vi "Get Required Objects.vi"(8 "error in":errorcluster, 11 "Device Profile in":refnum<class "Device Profile.lvclass">) -> (0 "error out":errorcluster, 2 "Required Objects":set{T1}(c389), 3 "Device Profile out":refnum<class "Device Profile.lvclass">)   [LabVIEW 2020, in "CANopen.lvlib" / "Device Profile.lvclass"]
uses:
  Device Profile.lvclass
  Device Profile.lvclass/Device Profile.ctl
  Typedefs/Data Type.ctl
  CANopen.lvlib
  Typedefs/OD Entry Spec.ctl
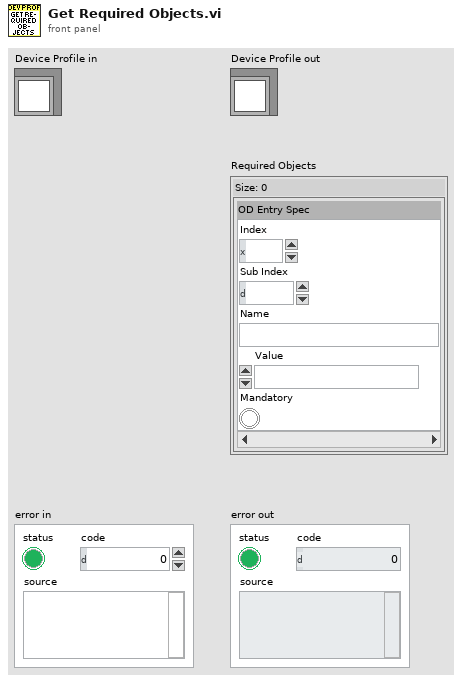
[diagram p1: front panel]
types:
  T1 = typedef "CANopen.lvlib/OD Entry Spec.ctl" = cluster{"Index":u16, "Sub Index":u8, "Name":string, "Value":T2, "Mandatory":bool}
  T2 = typedef "CANopen.lvlib/Data Type.ctl" = u16
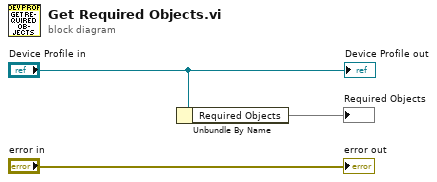
[diagram p0: block diagram]
diagram:
  n1 = Unbundle By Name("Device Profile in") -> ("Required Objects"=→"Required Objects":set{T1})
  "error out" <- "error in"
  "Device Profile out" <- "Device Profile in"
